vi "Trajectory_SampleReverse.vi"(9 "Time":dbl, 11 "InputTRAJECTORY":T5 {"TotalTImeSecs" format="%20.3f"}) -> (3 "OutputTRAJ_STATE":T1={"TimeSeconds"=0.0, "Velocity"=0.0, "Acceleration"=0.0, "POSE"={"TRANSLATION"={"X"=0.0, "Y"=0.0}, "ROTATION"={"VALUE"=0.0, "COS"=1.0, "SIN"=0.0}}, "Curvature"=0.0})   [LabVIEW 2019, in "Trajectory_Library.lvlib"]
doc: "Sample the trajectory at a point in time. The trajectory is sampled in reverse such that the ending time becomes 0 and the beginning time is the maximum time. The selected trajectory state is then transformed to be relative to end of the trajectory.\n\nThis routine does not exist in WPILIB\n \nParameters:\n - InputTrajectory - The Trajectory data structure\n - time - The point in time since the beginning of the trajectory to sample. (seconds)\n\nReturns:\n - OutputTrajState - The state at that point in time."
uses:
  Trajectory_Library.lvlib
  TRAJECTORY.ctl
  TRAJ_STATE.ctl
  POSE2D.ctl
  TRANSLATION2D.ctl
  ROTATION2D.ctl
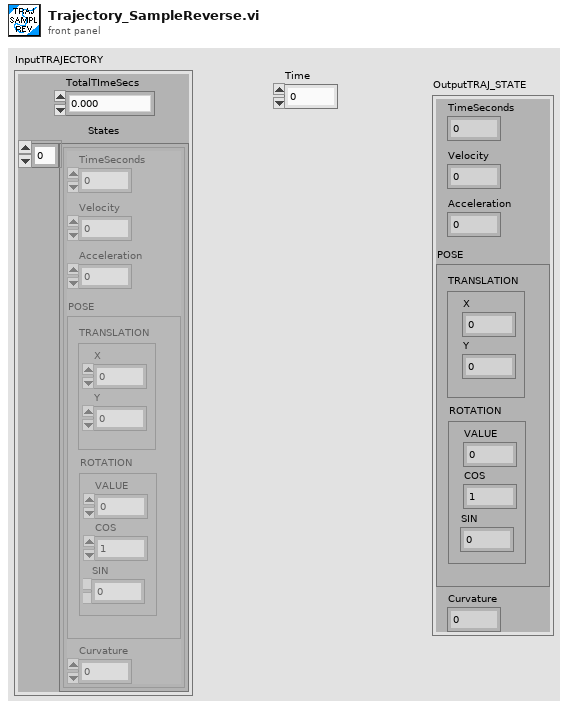
[diagram p1: front panel]
types:
  T1 = typedef "Trajectory_Library.lvlib/TRAJ_STATE.ctl" = cluster{"TimeSeconds":dbl, "Velocity":dbl, "Acceleration":dbl, "POSE":T2, "Curvature":dbl}
  T2 = typedef "Trajectory_Library.lvlib/POSE2D.ctl" = cluster{"TRANSLATION":T3, "ROTATION":T4}
  T3 = typedef "Trajectory_Library.lvlib/TRANSLATION2D.ctl" = cluster{"X":dbl, "Y":dbl}
  T4 = typedef "Trajectory_Library.lvlib/ROTATION2D.ctl" = cluster{"VALUE":dbl, "COS":dbl, "SIN":dbl}
  T5 = typedef "Trajectory_Library.lvlib/TRAJECTORY.ctl" = cluster{"TotalTImeSecs":dbl, "States":T1[]}
  T6 = typedef "Trajectory_Library.lvlib/TRANSFORM2D.ctl" = cluster{"TRANSLATION":T3, "ROTATION":T4}
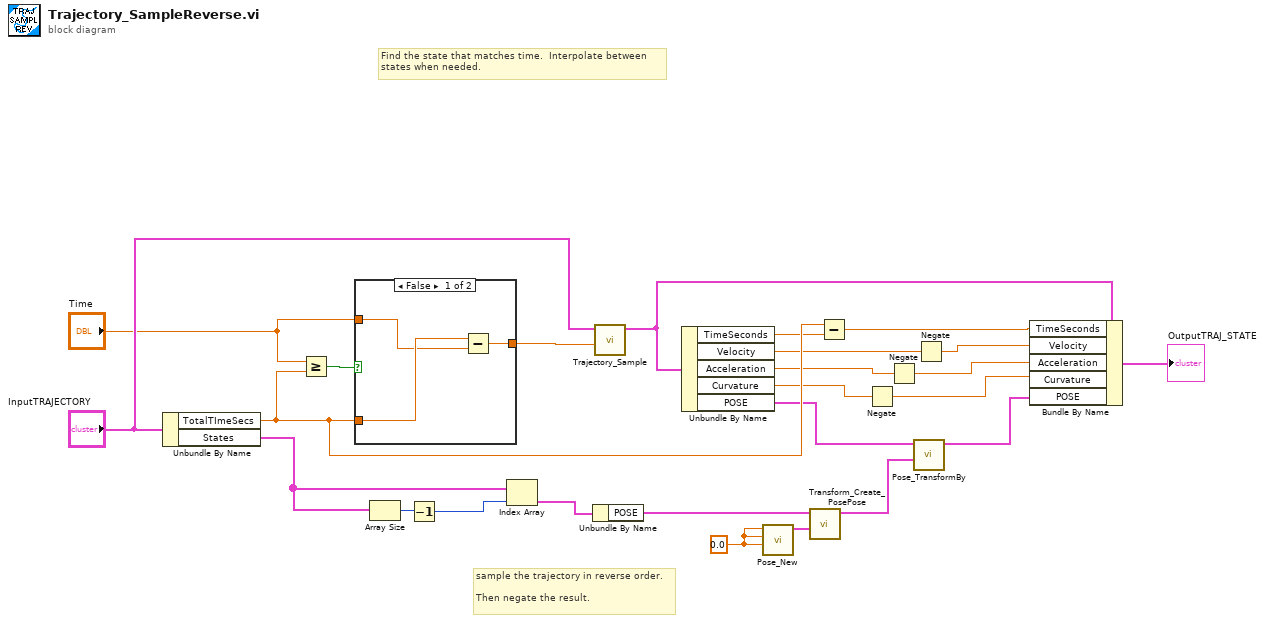
[diagram p0: block diagram]
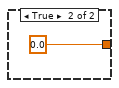
[diagram p2: hidden frame]
diagram:
  w9 = 0.0 ("X")
  # "sample the trajectory in reverse order.\n\nThen negate the result."
  # "Find the state that matches time.  Interpolate between\nstates when needed."
  n1 = Unbundle By Name("InputTRAJECTORY") -> ("TotalTImeSecs"=w19:dbl, "States"=w21:T1[])
  n2 = Greater Or Equal?(x="Time", y=w19) -> (x >= y?=w25:bool)
  n3 = case shown="False" w25 {
    tunnel: [w26 0.0] -> w2
    tunnel: w19 -> [w28 _]
    tunnel: "Time" -> [w27 _]
    frame False {
      n4 = Subtract(x=w28, y=w27) -> (x-y=w26:dbl)
    }
    frame True {
    }
  }
  n5 = Array Size(array=w21) -> (size(s)=w23:i32)
  n6 = Decrement(x=w23) -> (x-1=w22:i32)
  n7 = Index Array(array=w21, index=w22) -> (element=w8:T1)
  n8 = Unbundle By Name(w8) -> ("POSE"=w7:T2)
  n9 = call "Trajectory_Sample.vi"("Time"=w2, "InputTRAJECTORY"="InputTRAJECTORY") -> ("OutputTRAJ_STATE"=w20:T1)  [unwired: 9 in]
  n10 = Unbundle By Name(w20) -> ("TimeSeconds"=w18:dbl, "Velocity"=w16:dbl, "Acceleration"=w14:dbl, "Curvature"=w13:dbl, "POSE"=w5:T2)
  n11 = call "Pose_New.vi"("Heading"=w9, "Y"=w9, "X"=w9) -> ("out POSe"=w10:T2)  [unwired: 8 in]
  n12 = call "Transform_Create_PosePose.vi"("last POSE"=w10, "initial POSE"=w7) -> ("TRANSFORM"=w6:T6)  [unwired: 9 in]
  n13 = Subtract(x=w19, y=w18) -> (x-y=w17:dbl)
  n14 = Negate(x=w13) -> (-x=w11:dbl)
  n15 = Negate(x=w14) -> (-x=w12:dbl)
  n16 = call "Pose_TransformBy.vi"("other TRANSFORM"=w6, "in POSE"=w5) -> ("out POSE"=w4:T2)  [unwired: 9 in]
  n17 = Negate(x=w16) -> (-x=w15:dbl)
  n18 = Bundle By Name(cluster=w20, "TimeSeconds"=w17, "Velocity"=w15, "Acceleration"=w12, "Curvature"=w11, "POSE"=w4) -> (→"OutputTRAJ_STATE":T1)
